vi "Counts Update.vi"(5 "Perf":T1, 6 "output cluster":T4, 7 "Cluster":T3, 8 "Desired Cycle Time (s)":dbl=2.0, 9 "Previous Run Time":dbl, 10 "Parts Count":u32, 11 "Counts in":cluster{"OutputCount":u32, "RejectCount":u32}) -> (0 "Run Time":dbl, 1 "OEE":T6={"AVL"=100.0, "PRF"=100.0, "QUA"=100.0, "OEE"=0.0} {"OEE" format="%#.1f"; "QUA" min=0.0 max=100.0 step=0.1; "PRF" min=0.0 max=100.0 step=0.1; "AVL" min=0.0 max=100.0 step=0.1}, 2 "Auto Stats":T5={"Time"=timestamp(0 s since 1904-01-01), "OEE"={"AVL"=100.0, "PRF"=100.0, "QUA"=100.0, "OEE"=0.0}, "Auto Times"={"Index Time"=0, "TF Time"=0, "Insertion Time"=0, "Cutting Time"=0, "PF Time"=0, "Meas. Time"=0, "Reject Time"=0}, "Counts out"={"OutputCount"=0, "RejectCount"=0}, "Measurements"={"1"=0.0, "2"=0.0, "3"=0.0, "4"=0.0}, "Outputs"={"OutputCount"=0, "Numeric Control"=0}} {"OEE"."OEE" format="%#.1f"; "OEE"."QUA" min=0.0 max=100.0 step=0.1; "OEE"."PRF" min=0.0 max=100.0 step=0.1; "OEE"."AVL" min=0.0 max=100.0 step=0.1}, 3 "Counts out":cluster{"OutputCount":u32, "RejectCount":u32})   [LabVIEW 2017]
uses:
  support/Controls/Auto Stats.ctl
  Controls/Auto Times.ctl
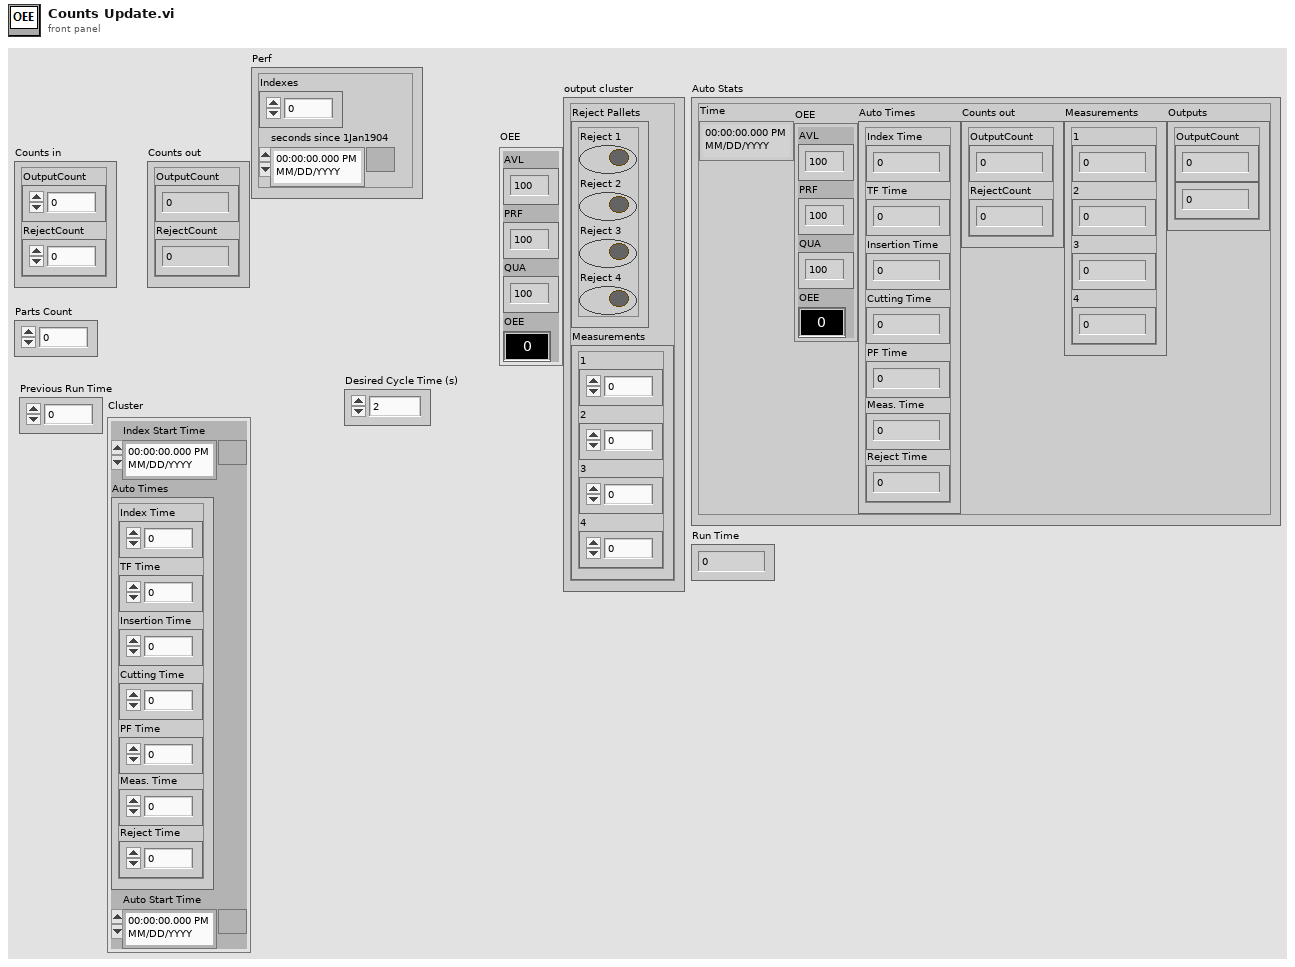
[diagram p1: front panel]
types:
  T1 = cluster{"Indexes":i32, "seconds since 1Jan1904":timestamp}
  T2 = typedef "Auto Times.ctl" = cluster{"Index Time":u32, "TF Time":u32, "Insertion Time":u32, "Cutting Time":u32, "PF Time":u32, "Meas. Time":u32, "Reject Time":u32}
  T3 = cluster{"Index Start Time":timestamp, "Auto Times":T2, "Auto Start Time":timestamp}
  T4 = cluster{"Reject Pallets":cluster{"Reject 1":bool, "Reject 2":bool, "Reject 3":bool, "Reject 4":bool}, "Measurements":cluster{"1":dbl, "2":dbl, "3":dbl, "4":dbl}}
  T5 = typedef "Auto Stats.ctl" = cluster{"Time":timestamp, "OEE":cluster{"AVL":dbl, "PRF":dbl, "QUA":dbl, "OEE":dbl}, "Auto Times":T2, "Counts out":cluster{"OutputCount":u32, "RejectCount":u32}, "Measurements":cluster{"1":dbl, "2":dbl, "3":dbl, "4":dbl}, "Outputs":cluster{"OutputCount":u32, "Numeric Control":u32}}
  T6 = cluster{"AVL":dbl, "PRF":dbl, "QUA":dbl, "OEE":dbl}
  T7 = cluster{"Reject 1":bool, "Reject 2":bool, "Reject 3":bool, "Reject 4":bool}
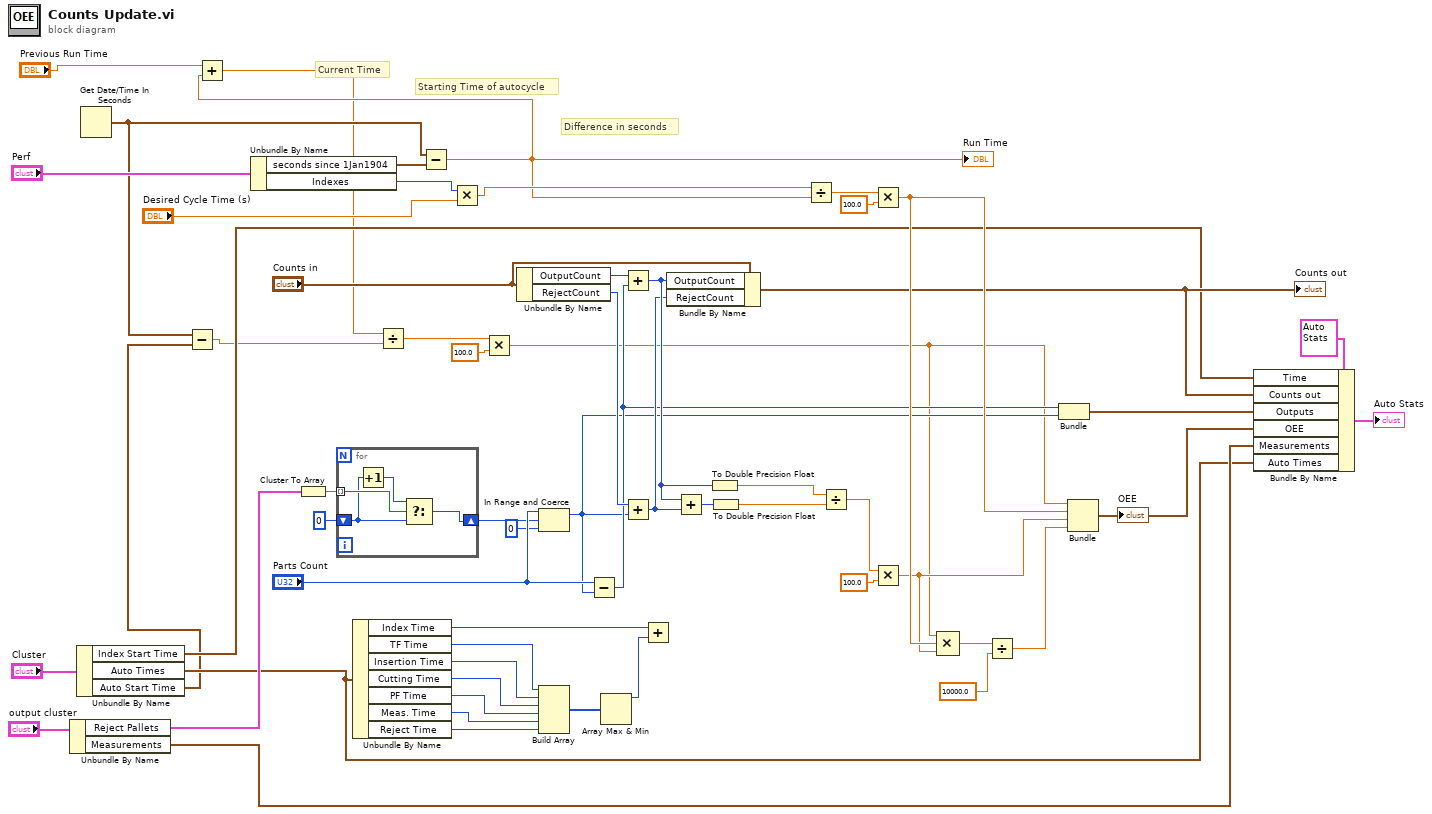
[diagram p0: block diagram]
diagram:
  # "Difference in seconds"
  # "Starting Time of autocycle"
  # "Current Time"
  n1 = Unbundle By Name("output cluster") -> ("Reject Pallets"=w23:T7, "Measurements"=w24:cluster{"1":dbl, "2":dbl, "3":dbl, "4":dbl})
  n2 = Unbundle By Name("Cluster") -> ("Index Start Time"=w20:timestamp, "Auto Times"=w21:T2, "Auto Start Time"=w7:timestamp)
  n3 = Get Date/Time In Seconds() -> (seconds since 1Jan1904=w9:timestamp)
  n4 = Subtract(x=w9, y=w7) -> (x-y=w5:dbl)
  n5 = Unbundle By Name("Perf") -> ("seconds since 1Jan1904"=w18:timestamp, "Indexes"=w16:i32)
  n6 = Cluster To Array(cluster=w23) -> (array=w56:bool[])
  n7 = for {
    tunnel: w56 -> [w62] mode=indexing
    shift-right: [w61] -> w11
    shift-left: u32 0 -> [w60]
    n8 = Increment(x=w60) -> (x+1=w59:u32)
    n9 = Select(t=w59, s=w62, f=w60) -> (s? t:f=w61:u32)
  }
  n10 = Unbundle By Name(w21) -> ("Index Time"=w47:u32, "TF Time"=w41:u32, "Insertion Time"=w42:u32, "Cutting Time"=w43:u32, "PF Time"=w44:u32, "Meas. Time"=w45:u32, "Reject Time"=w46:u32)
  n11 = Subtract(x=w9, y=w18) -> (x-y=w3:dbl)
  "Run Time" <- w3
  n12 = Add(x="Previous Run Time", y=w3) -> (x+y=w2:dbl)
  n13 = Divide(x=w2, y=w5) -> (x/y=w1:dbl)
  n14 = Multiply(x=w16, y="Desired Cycle Time (s)") -> (x*y=w15:dbl)
  n15 = Multiply(x=w1, y=100.0) -> (x*y=w6:dbl)
  n16 = Unbundle By Name("Counts in") -> ("OutputCount"=w58:u32, "RejectCount"=w57:u32)
  n17 = In Range and Coerce(upper limit="Parts Count", x=w11, lower limit=u32 0) -> (coerced(x)=w10:u32)  [unwired: 1 out]
  n18 = Build Array(w41, w42, w43, w44, w45, w46) -> (w40:u32[])
  n19 = Subtract(x="Parts Count", y=w10) -> (x-y=w14:u32)
  n20 = Array Max & Min(array=w40) -> (max value=w39:u32)  [unwired: 3 out]
  n21 = Add(x=w58, y=w14) -> (x+y=w52:u32)
  n22 = Add(x=w57, y=w10) -> (x+y=w31:u32)
  n23 = Add(x=w47, y=w39) -> ()  [unwired: 1 out]
  n24 = Bundle By Name(cluster="Counts in", "OutputCount"=w52, "RejectCount"=w31) -> (w27:cluster{"OutputCount":u32, "RejectCount":u32})
  "Counts out" <- w27
  n25 = Add(x=w52, y=w31) -> (x+y=w53:u32)
  n26 = To Double Precision Float(number=w52) -> (double precision float=w33:dbl)
  n27 = To Double Precision Float(number=w53) -> (double precision float=w32:dbl)
  n28 = Divide(x=w15, y=w3) -> (x/y=w37:dbl)
  n29 = Divide(x=w33, y=w32) -> (x/y=w50:dbl)
  n30 = Multiply(x=w37, y=100.0) -> (x*y=w35:dbl)
  n31 = Multiply(x=w50, y=100.0) -> (x*y=w34:dbl)
  n32 = Compound Arithmetic op=MULTIPLY(w6, w35, w34) -> (w51:dbl)
  n33 = Divide(x=w51, y=10000.0) -> (x/y=w36:dbl)
  n34 = Bundle(w14, "Parts Count"=w10) -> (w29:cluster{u32, "Parts Count":u32})  [unwired: 1 in]
  n35 = Bundle(w6, w35, w34, w36) -> (w28:cluster{dbl, dbl, dbl, dbl})  [unwired: 1 in]
  "OEE" <- w28
  n36 = Bundle By Name(cluster=T5 {"Time"=timestamp(0 s since 1904-01-01), "OEE"={"AVL"=100.0, "PRF"=100.0, "QUA"=100.0, "OEE"=0.0}, "Auto Times"={"Index Time"=0, "TF Time"=0, "Insertion Time"=0, "Cutting Time"=0, "PF Time"=0, "Meas. Time"=0, "Reject Time"=0}, "Counts out"={"OutputCount"=0, "RejectCount"=0}, "Measurements"={"1"=0.0, "2"=0.0, "3"=0.0, "4"=0.0}, "Outputs"={"OutputCount"=0, "Numeric Control"=0}} ("Auto Stats"), "Time"=w20, "Counts out"=w27, "Outputs"=w29, "OEE"=w28, "Measurements"=w24, "Auto Times"=w21) -> (→"Auto Stats":T5)
